vi "Terminal-DriverSystem-SelfCheck.vi"(8 "error in (no error)":errorcluster caption="错误输入（无错误）") -> (0 "error out":errorcluster caption="错误输出")   [LabVIEW 2014]
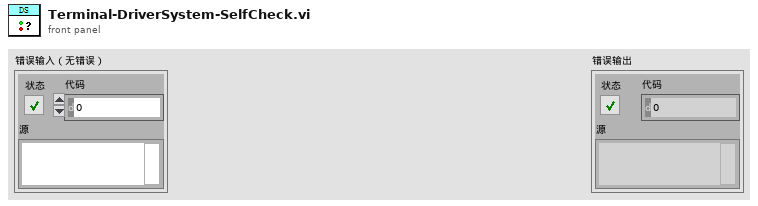
[diagram p1: front panel]
types:
  T1 = cluster{"变送器配电模块电压":u16, "变频器电流":u16, "变频器电压":u16, "变频器频率":u16, "动力子系统状态字":cluster{"电机温度过高报警":bool, "变频器电气参数异常报警":bool, "电机过载报警":bool, "电机转速误差过大报警":bool}}
  T2 = cluster{"电机温度过高报警":bool, "变频器电气参数异常报警":bool, "电机过载报警":bool, "电机转速误差过大报警":bool}
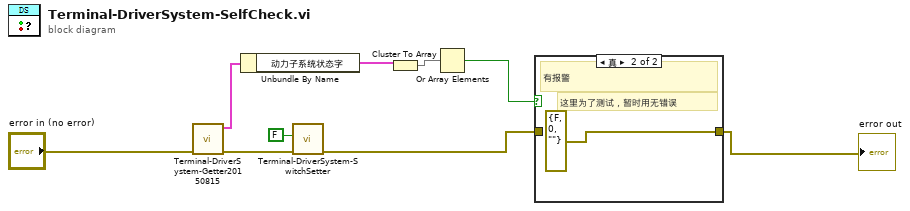
[diagram p0: block diagram]
diagram:
  n1 = call "Terminal-DriverSystem-Getter20150815.vi"("error in (no error)"="error in (no error)") -> ("error out"=w8:errorcluster, "设备信息"=w6:T1)  [unwired: 8 in, 1 out]
  n2 = Unbundle By Name(w6) -> ("动力子系统状态字"=w5:T2)
  n3 = call "Terminal-DriverSystem-SwitchSetter.vi"("error in (no error)"=w8, "启停"=FALSE) -> ("error out"=w2:errorcluster)  [unwired: 9 in]
  n4 = Cluster To Array(cluster=w5) -> (array=w4:bool[])
  n5 = Or Array Elements(Boolean array=w4) -> (logical OR=w3:bool)
  n6 = case shown="真" w3 {
    tunnel: [w10 errorcluster {"status"=FALSE, "code"=0, "source"=""} ("错误常量")] -> w1
    tunnel: w2 -> [w10 _]
    frame False {
      # "没有报警"
    }
    frame True {
      # "这里为了测试，暂时用无错误"
      # "有报警"
    }
  }
  "error out" <- w1
